vi "Read Parent Fully Qualified Name.vi"(11 "UniqueName in":refnum<class "UniqueName.lvclass">) -> (2 "Parent Fully Qualified Name":string, 3 "UniqueName out":refnum<class "UniqueName.lvclass">)   [LabVIEW 2014, in "UniqueName.lvlib" / "UniqueName.lvclass"]
uses:
  UniqueName.lvclass
  UniqueName.lvclass/UniqueName.ctl
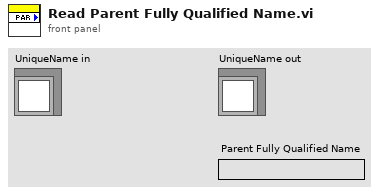
[diagram p1: front panel]
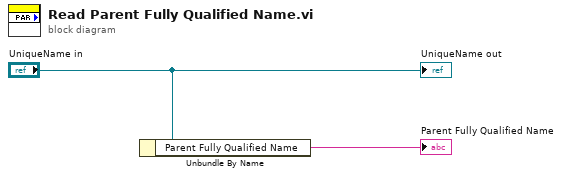
[diagram p0: block diagram]
diagram:
  n1 = Unbundle By Name("UniqueName in") -> ("Parent Fully Qualified Name"=→"Parent Fully Qualified Name":string)
  "UniqueName out" <- "UniqueName in"
